vi "LibXML_FirstMatchNode.vi"(8 "error in":errorcluster, 9 "queryString":string, 10 "root node":u32, 11 "doc":u32) -> (0 "error out":errorcluster, 2 "Matched Node":u32, 3 "doc out":u32)   [LabVIEW 2019, in "Tools.lvlib"]
doc: "Gets the first node that matches the XPath"
uses:
  Tools.lvlib
  libxml2/LibXML_QueryXPathExpr.vi
  libxml2/LibXML_GetNumberOfNodes.vi
  Error Cluster From Error Code_subroutine.vi
  <vilib>/Utility/error.llb/Trim Whitespace.vi
  LibXML.lvlib
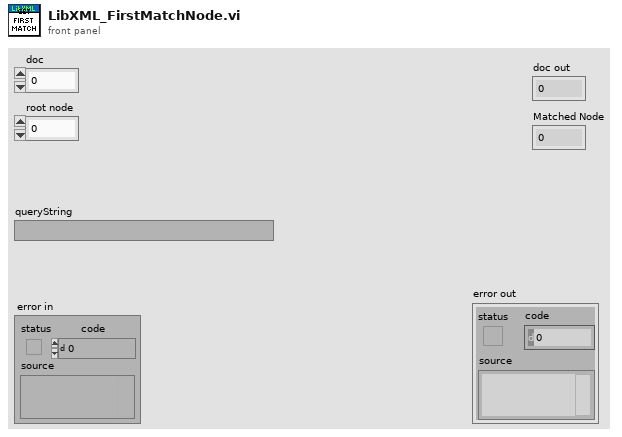
[diagram p1: front panel]
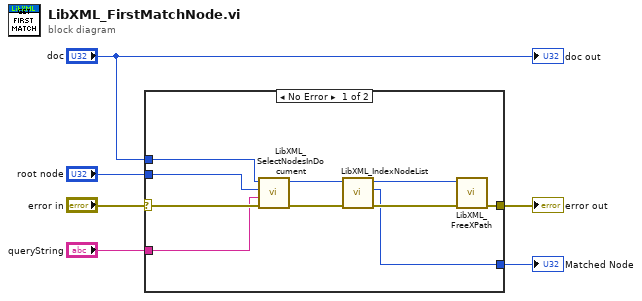
[diagram p0: block diagram]
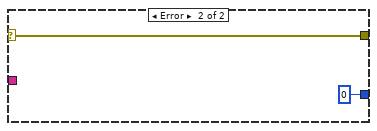
[diagram p2: hidden frame]
diagram:
  n1 = case shown="No Error" "error in" {
    selector: "error in" -> [w11 w18]
    tunnel: [w9 u32 0 ("NodePtr")] -> w3
    tunnel: [w12 w18] -> w6
    tunnel: "queryString" -> [w10 _]
    tunnel: "doc" -> [w8 _]
    tunnel: "root node" -> [w7 _]
    frame No Error {
      n2 = call "LibXML_SelectNodesInDocument.vi"("error in"=w11, "queryString"=w10, "rootnode (root of doc)"=w7, "doc"=w8) -> ("error out"=w13:errorcluster, "xmlXPathObj"=w14:u32)  [unwired: 2 in, 4 out]
      n3 = call "LibXML_IndexNodeList.vi"("error in"=w13, "XPathObj"=w14) -> ("error out"=w15:errorcluster, "NodePtr"=w9:u32, "XPathObj out"=w16:u32)  [unwired: 7 in]
      n4 = call "LibXML_FreeXPath.vi"("error in"=w15, "XPathObj"=w16) -> ("error out"=w12:errorcluster)  [unwired: 9 in]
    }
    frame Error {
    }
  }
  "error out" <- w6
  "Matched Node" <- w3
  "doc out" <- "doc"
